vi "LoadPressureAndTangents XYGraph.vi"(4 "error in (no error)":errorcluster, 5 "Red Graph":refnum<vi>, 6 "ResetFrontImage":bool, 7 "Blue Graph":refnum<vi>) -> (0 "error out":errorcluster, 3 "output cluster":cluster{dbl, dbl, dbl, dbl})   [LabVIEW 2013, in "main.lvlib"]
uses:
  main.lvlib
  Controls/Enum Process Data.ctl
  Controls/Combobox Filename.ctl
  Controls/Enum Variables.ctl
  <userlib>/_OpenG.lib/file/file.llb/File Exists - Scalar__ogtk.vi
  <vilib>/Utility/file.llb/Read From Spreadsheet File (DBL).vi
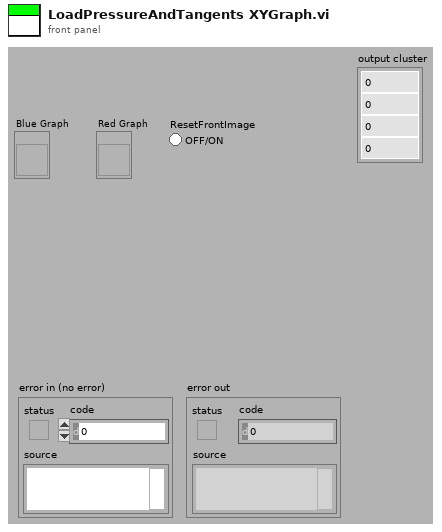
[diagram p1: front panel]
types:
  T1 = typedef "main.lvlib/Enum Variables.ctl" = enum16{"SetAcqFilter", "GetAcqFilter", "Set Filter", "Get Filter", "Set Height", "Get Height", "Set Blue Pressure", "Get Blue Pressure", "Set Red Pressure", "Get Red Pressure", "Init", "Reset Pressure", "Set Red Cursors", "Get Red Cursors", "Set Blue Cursors", "Get Blue Cursors", "Set Language", "Get Language", "Set Active Graphs", "Get ActiveGraphs", "Set Method", "Get Method", "Set Encryption", "Get Encryption", "Set ExcelVersion", "Get ExcelVersion", "Set DICOM Avail", "Get DICOM Avail", "Set DICOM Encode", "Get DICOM Encode", "Set JournalExport", "Get JournalExport", "Set Sequence", "Get Sequence", "Set DAQ Connected", "Get DAQ Connected", "Set Current Graph", "Get Current Graph", "Set General Settings", "Get Hyphenation", "Set Arm Calc Method", "Get Arm Calc Method", "Set Dicom Tags", "Get Dicom Tags", "Set BT Serial", "Get BT Serial", "Set BT Accepted Serials", "Get BT Accepted Serials", "Get BT License", "Set BT License"}
  T2 = typedef "main.lvlib/Combobox Filename.ctl" = string
  T3 = typedef "main.lvlib/Enum Process Data.ctl" = enum16{"Init", "Set Cursor Mode", "Set Data Path", "Get All"}
  T4 = cluster{dbl, dbl, "Armpressure":dbl, "Armpressure":dbl}
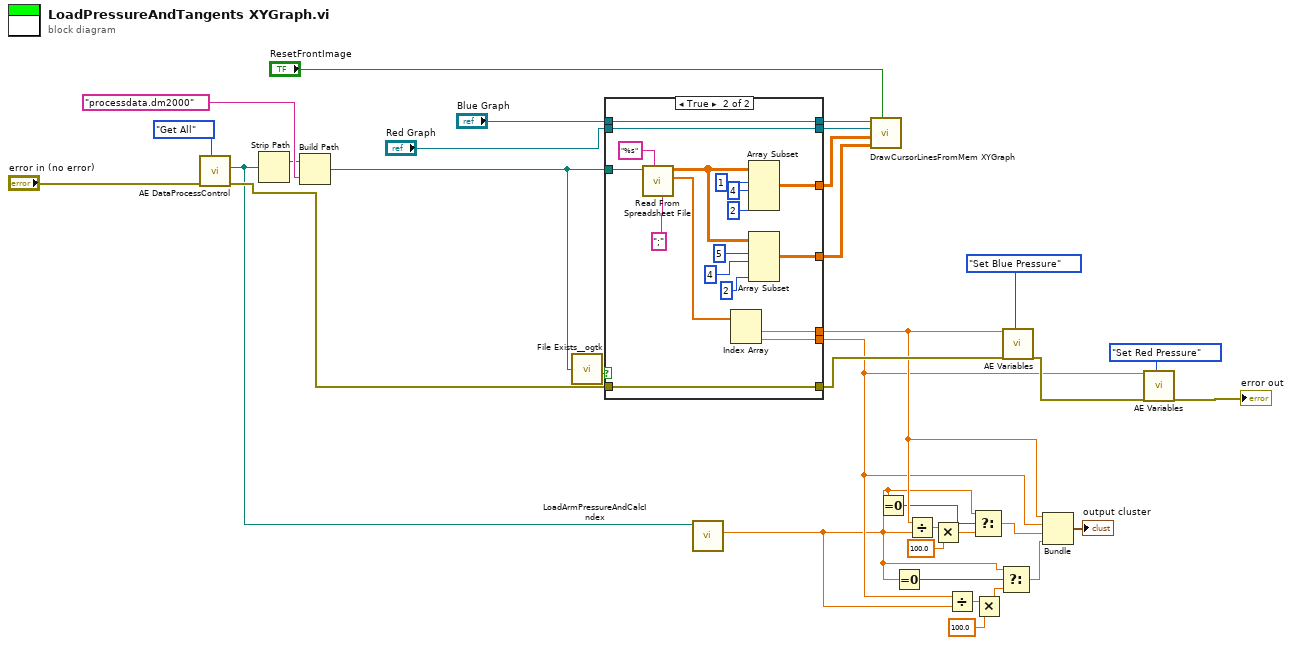
[diagram p0: block diagram]
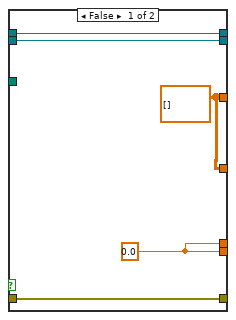
[diagram p2: hidden frame]
diagram:
  n1 = call "AE DataProcessControl.vi"("Action"=Enum_Process_Data."Get All", "error in (no error)"="error in (no error)") -> ("error out"=w20:errorcluster, "Data Path Out"=w16:path)  [unwired: 7 in, 1 out]
  n2 = Strip Path(path=w16) -> (stripped path=w23:path)  [unwired: 1 out]
  n3 = Build Path(base path=w23, name or relative path=T2 "processdata.dm2000" ("FileName")) -> (appended path=w34:path)
  n4 = call-poly <userlib>:"File Exists__ogtk.vi"("file path"=w34) -> ("exists"=w29:bool)  [unwired: 6 in, 1 out]
  n5 = case shown="True" w29 {
    tunnel: w34 -> [_ w54]
    tunnel: [w39 w53] -> w10
    tunnel: [w39 w52] -> w13
    tunnel: [w38 w48] -> w27
    tunnel: [w38 w46] -> w28
    tunnel: [w37 w42] -> w31
    tunnel: "Blue Graph" -> [w37 w42]
    tunnel: "Red Graph" -> [w36 w41]
    tunnel: [w36 w41] -> w32
    tunnel: w20 -> [w35 w40]
    tunnel: [w35 w40] -> w19
    frame False {
      w38 = dbl[][] []
      w39 = 0.0
    }
    frame True {
      n6 = call-poly <vilib>:"Read From Spreadsheet File.vi"("delimiter (\\t)"=";" ("delimiter (\\t)"), "format (%.3f)"="%s", "file path (dialog if empty)"=w54) -> ("first row"=w55:dbl[], "all rows"=w47:dbl[][])  [unwired: 4 in, 3 out]
      n7 = Index Array(array=w55) -> (element #1=w52:dbl, element #2=w53:dbl)  [unwired: 2 in]
      n8 = Array Subset(array=w47, index (row)=1 ("index"), length (row)=4 ("length"), length (col)=2 ("length")) -> (w48:dbl[][])  [unwired: 1 in]
      n9 = Array Subset(array=w47, index (row)=5 ("index"), length (row)=4 ("length"), length (col)=2 ("length")) -> (w46:dbl[][])  [unwired: 1 in]
    }
  }
  n10 = call "LoadArmPressureAndCalcIndex.vi"("Path"=w16) -> ("Armpressure"=w3:dbl)  [unwired: 8 in, 2 out]
  n11 = call "DrawCursorLinesFromMem XYGraph.vi"("CursorMode"="ResetFrontImage", "RedPositionArray"=w28, "BluePositionArray"=w27, "Red"=w32, "Blue"=w31) -> ()  [unwired: 7 in]
  n12 = Equal To 0?(x=w3) -> (x = 0?=w8:bool)
  n13 = Equal To 0?(x=w3) -> (x = 0?=w5:bool)
  n14 = Divide(x=w13, y=w3) -> (x/y=w15:dbl)
  n15 = Multiply(x=w15, y=100.0) -> (x*y=w7:dbl)
  n16 = Divide(x=w10, y=w3) -> (x/y=w12:dbl)
  n17 = Select(t=w3, s=w8, f=w7) -> (s? t:f=w6:dbl)
  n18 = Multiply(x=w12, y=100.0) -> (x*y=w4:dbl)
  n19 = Select(t=w3, s=w5, f=w4) -> (s? t:f=w2:dbl)
  n20 = call "AE Variables.vi"("VariantIn"=w13, "error in (no error)"=w19, "Action"=Enum_Variables."Set Blue Pressure") -> ("error out"=w18:errorcluster)  [unwired: 9 in, 7 out]
  n21 = Bundle(w13, w10, "Armpressure"=w6, "Armpressure"=w2) -> (→"output cluster":T4)  [unwired: 1 in]
  n22 = call "AE Variables.vi"("VariantIn"=w10, "error in (no error)"=w18, "Action"=Enum_Variables."Set Red Pressure") -> ("error out"=→"error out":errorcluster)  [unwired: 9 in, 7 out]
